vi "DMA Example with Size Distribution.vi"() -> ()   [LabVIEW 2014]
uses:
  Atmospheric/Atmospheric Constants.vi
  Atmospheric/Atmospheric Library.lvlib
  <vilib>/gmath/NI_Gmath.lvlib
panel:
  out "V":dbl
  in  "Number Concentration":dbl=20000.0
  in  "Standard Dev":dbl=2.0
  in  "Geometric Mean":dbl=0.1
  in  "Selected Size":dbl=0.3
  in  "# of Charges":i32=4
  in  "T (C)":dbl=20.0
  in  "P (mb)":dbl=850.0
  in  "Qaerosol":dbl=1.5
  in  "Qsample":dbl=1.5
  in  "Qsheath":dbl=10.0
  in  "Qexcess":dbl=10.0
  out "Distribution":cluster{dbl[], dbl[]}[](graph)
  # "Distribution Parameters"
  # "Size Selection"
  # "Ambient \nConditions"
  # "Flow Rates in LPM"
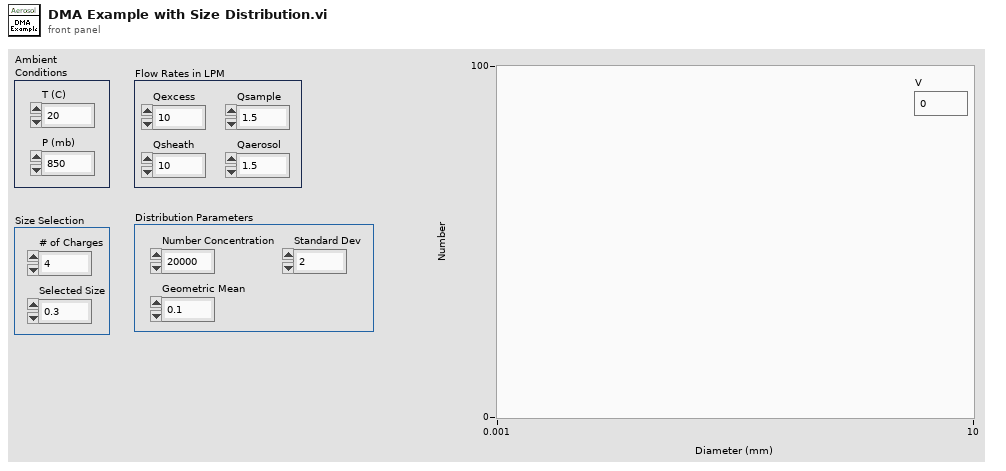
[diagram p1: front panel]
types:
  T1 = cluster{"Omega":dbl[], "dP*Zstar":dbl[], "Zstar":dbl[]}
  T2 = cluster{"Charge":i32, "D (mm)":dbl, "Cc":dbl, "f":dbl}[]
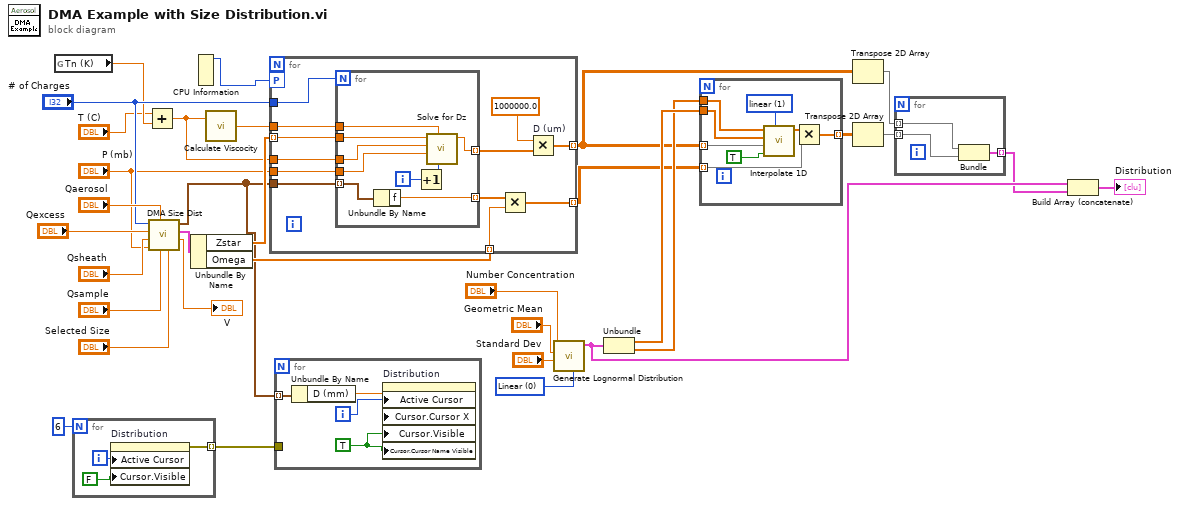
[diagram p0: block diagram]
diagram:
  w31 = u16 0 items=["Linear", "Logarithmic"] ("type")
  n1 = global read "Atmospheric Constants.vi" "Tn (K)"() -> (w23:dbl)
  n2 = for {
    N: 6 -> [_]
    tunnel: [w34] -> w4 mode=indexing
    i -> [w36]
    n3 = property on="Distribution" class="XYGraph (strict)"("Active Cursor"=w36, "Cursor.Visible"=FALSE) -> (error out=w34:errorcluster)  [unwired: 2 in, 1 out]
  }
  n4 = Add(x="T (C)", y=w23) -> (x+y=w7:dbl)
  n5 = call "DMA Size Dist.vi"("Selected Size"="Selected Size", "Qsample"="Qsample", "Qaerosol"="Qaerosol", "P"="P (mb)", "Qsheath"="Qsheath", "Qexcess"="Qexcess", "# of Charges"="# of Charges") -> ("V"=→"V":dbl, "Omega Function"=w26:T1, "DMA Data Out"=w5:T2)  [unwired: 2 in]
  n6 = CPU Information() -> (4:w1:i32)  [unwired: 3 out]
  n7 = Unbundle By Name(w26) -> ("Zstar"=w25:dbl[], "Omega"=w10:dbl[])
  n8 = call "Calculate Viscocity.vi"("T(K)"=w7) -> ("mu (Pa*s)"=w22:dbl)  [unwired: 1 in]
  n9 = for {
    tunnel: w10 -> [w39] mode=indexing
    tunnel: w25 -> [w47] mode=indexing
    tunnel: "# of Charges" -> [w48]
    tunnel: w22 -> [w46]
    tunnel: w7 -> [w45]
    tunnel: "P (mb)" -> [w44]
    tunnel: w5 -> [w41]
    tunnel: [w38] -> w9 mode=indexing
    tunnel: [w37] -> w12 mode=indexing
    workers-P: w1 -> [_]
    n10 = for {
      N: w48 -> [_]
      tunnel: w47 -> [w56]
      tunnel: w46 -> [w55]
      tunnel: w45 -> [w54]
      tunnel: w44 -> [w53]
      tunnel: [w49] -> w43 mode=indexing
      tunnel: w41 -> [w51] mode=indexing
      tunnel: [w50] -> w40 mode=indexing
      i -> [w57]
      n11 = Unbundle By Name(w51) -> ("f"=w50:dbl)
      n12 = Increment(x=w57) -> (x+1=w52:i32)
      n13 = call "Solve for Dz.vi"("n"=w52, "mu"=w55, "P"=w53, "T"=w54, "Z1"=w56) -> ("dz"=w49:dbl)  [unwired: 5 in, 1 out]
    }
    n14 = Multiply(x=w40, y=w39) -> (x*y=w37:dbl[])
    n15 = Multiply "D (um)"(x=1000000.0, y=w43) -> (x*y=w38:dbl[])
  }
  n16 = for {
    tunnel: w5 -> [w60] mode=indexing
    tunnel: w4 -> [_]
    i -> [w61]
    w58 = TRUE
    n17 = Unbundle By Name(w60) -> ("D (mm)"=w59:dbl)
    n18 = property on="Distribution" class="XYGraph (strict)"("Active Cursor"=w61, "Cursor.Cursor X"=w59, "Cursor.Visible"=w58, "Cursor.Cursor Name Visible"=w58) -> ()  [unwired: 2 in, 2 out]
  }
  n19 = call "Generate Lognormal Distribution.vi"("type"=w31, "Standard Dev"="Standard Dev", "Geometric Mean"="Geometric Mean", "Number Concentration"="Number Concentration") -> ("Distribution"=w18:cluster{dbl[], dbl[]})  [unwired: 7 in]
  n20 = Unbundle(w18) -> (w20:dbl[], w19:dbl[])
  n21 = for {
    tunnel: w20 -> [w69]
    tunnel: w19 -> [w68]
    tunnel: w9 -> [w67] mode=indexing
    tunnel: w12 -> [w63] mode=indexing
    tunnel: [w62] -> w13 mode=indexing
    w65 = 1 items=["nearest", "linear", "spline", "cubic Hermite", "Lagrange"] ("method")
    n22 = call <vilib>:"Interpolate 1D.vi"("method"=w65, "X is monotonic"=TRUE, "xi"=w67, "X"=w69, "Y"=w68) -> ("yi"=w64:dbl[])  [unwired: 4 in, 2 out]
    n23 = Multiply(x=w64, y=w63) -> (x*y=w62:dbl[])
  }
  n24 = Transpose 2D Array(2D array=w9) -> (transposed array=w11:dbl[][])
  n25 = Transpose 2D Array(2D array=w13) -> (transposed array=w14:dbl[][])
  n26 = for {
    tunnel: w14 -> [w71] mode=indexing
    tunnel: w11 -> [w70] mode=indexing
    tunnel: [w72] -> w15 mode=indexing
    n27 = Bundle(w70, w71) -> (w72:cluster{dbl[], dbl[]})  [unwired: 1 in]
  }
  n28 = Build Array (concatenate)(w18, w15) -> (→"Distribution":cluster{dbl[], dbl[]}[])
